vi "P_sat_correlation.vi"(1 "Unit":i16(ring)=1 items=["Kelvin", "Celcius"], 2 "Temperature":dbl) -> (0 "P Sat":dbl)   [LabVIEW 2015]
uses:
  <vilib>/express/express arith-compare/Formula/XNode/ExpressFormulaBlockNode.xnode
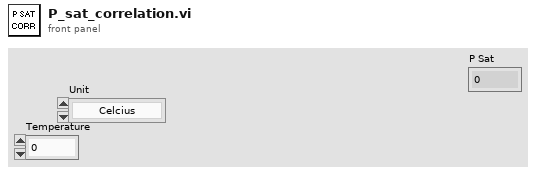
[diagram p1: front panel]
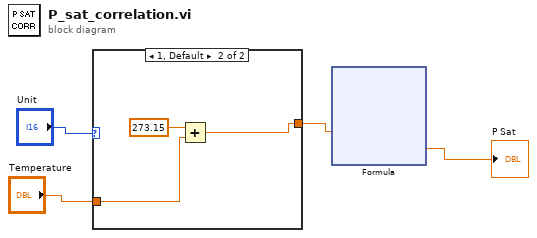
[diagram p0: block diagram]
diagram:
  n1 = case shown="1, Default" "Unit" {
    tunnel: "Temperature" -> [w5 w7]
    tunnel: [w5 w6] -> w2
    frame 0 {
    }
    frame 1, Default {
      n2 = Add(x=273.15, y=w7) -> (x+y=w6:dbl)
    }
  }
  n3 = xnode "Formula"("T"=w2) -> ("Result"=→"P Sat":dbl)  [unwired: 1 in, 1 out]
